vi "SIMCOMCommunicationTool_CF.vi"(0 "VISA资源名称":refnum<visa-resource-name>="COM26", 1 "MSComm":refnum<k7>, 2 "MEID":string, 5 "通信协议名称":string, 9 "DelayTime":u32=100, 11 "error in":errorcluster, 12 "Debug":bool=TRUE, 14 "Slot":T1) -> (3 "CMD":string="发送 重启:AT+CRESET\r反馈:\r\nOK\r\n\r\n", 4 "字符串数值":bool=TRUE, 6 "反馈结果":bool=TRUE, 10 "ReturnData":string, 15 "error out":errorcluster)   [LabVIEW 2013]
doc: "本范例根据用户指示，对串口执行读写操作。范例运行时可按下“写入”或“读取”按钮，以及修改“读数”。\n\n设置的串口参数必须匹配连接仪器或设备的参数。本范例中，“读数”参数可指定串口读取的字节数。如端口字节超过指定的字节数，超出部分将不会被读取。如端口字节数少于指定的字节数，将返回超时错误。\n\n本范例可扩展流控制选项以包括XON和XOFF，从而允许用户选择控制字符。同时，用户可启用或禁用中止符。部分设备需要通过终止符确定命令字符串的结束位置。部分设备将发送终止符以说明待读取数据的末端。本范例演示了缓冲区中检测到终止符时，结束“读取”操作或添加终止符至“写入”数据末端的方法。"
uses:
  SystemCode/SysControl/Slot.ctl
  <vilib>/Utility/NIReport.llb/NI_report.lvclass
  SourceCode/GlobalValue.vi
  <vilib>/Utility/error.llb/Error Cluster From Error Code.vi
  <vilib>/addons/_office/excel.llb/Excel Get Data ([str]).vi
  <vilib>/ErrorRing/Error Ring.xnode
  <vilib>/addons/_office/NI_ReportGenerationToolkit.lvlib
  <vilib>/Utility/NIReport.llb/Excel/NI_Excel.lvclass
panel:
  out "Data":string[][](array[string])=[["8986031490021881534", "460036161669975", "2A645416CB435F94", "8006A127", "460036161669975@mycdma.cn", "DB60264368A1D188", "18101891253", "A1000021A59070"], ["8986031490021881535", "460036161669976", "32FA5764D69C76BE", "80FAE4E6", "460036161669976@mycdma.cn", "B3AA1B3D2F0D5593", "18964872399", "A1000021A58D61"], ["", "", "", "", "", "", "", ""], ["", "", "", "", "", "", "", ""], ["", "", "", "", "", "", "", ""], ["", "", "", "", "", "", "", ""], ["", "", "", "", "", "", "", ""], ["", "", "", "", "", "", "", ""], ["", "", "", "", "", "", "", ""], ["", "", "", "", "", "", "", ""], ["", "各位，模块烧号主要是写五码，包括IMSI、AKEY、MEID（ESN）、AN(EVDO USER)、AAA(EVDO PWD)。", "", "", "", "", "", ""], ["", "其中ESN和MEID在模块出厂时已经写入，两者均可通过AT指令读取，但ESN不可更改。", "", "", "", "", "", ""], ["", "经询问及实际测试，上海电信绑定ESN号而广东电信未绑定，意味着上海电信五码烧录到其它模块是不可用的，但广东电信则无此限制。", "", "", "", "", "", ""], ["", "", "", "", "", "", "", ""], ["", "", "", "", "", "", "", ""], ["", "目前已确定跟上海电信合作，后续模块及卡号使用过程中，如遇到模块损坏，则意味着该卡必须销号（除非向电信申请绑定新的ESN），否则烧录到其它模块中是没用的。", "", "", "", "", "", ""]]
  in  "命令列表":u16(ring)=18 items=["查询RTRECF", "设置RTRECF", "查询MEID", "设置MEID", "查询ESN", "设置ESN", "查询AKEY", "设置AKEY", "查询IMSI1", "设置IMSI1", "查询IMSI2", "设置IMSI2", "查询IMSI3", "设置IMSI3", "设置EVDO账号", "设置EVDO密码", "打开音频LOOPBACK", "关闭音频LOOPBACK", "重启", "打开网络", "查询网络状态", "连网测试", "查询CIP", "切换声音通道", "测试登录", "拨号", "挂断", "查询IP", "AT+CSOCKAUTHNV", "AT+CSOCKAUTH", "查询2G信号", "查询3G信号", "H330测试通讯", "H330打开音频回环", "H330关闭音频回环", "H330拨号"]
  out "ConfigPath":string="D:\\导航\\T-BOX\\新建文件夹\\config\\通信协议.xls"
  out "DataType":string="AT+CRESET"
  out "命令":string="AT+CRESET\r"
  out "响应":string="\r\nOK\r\n"
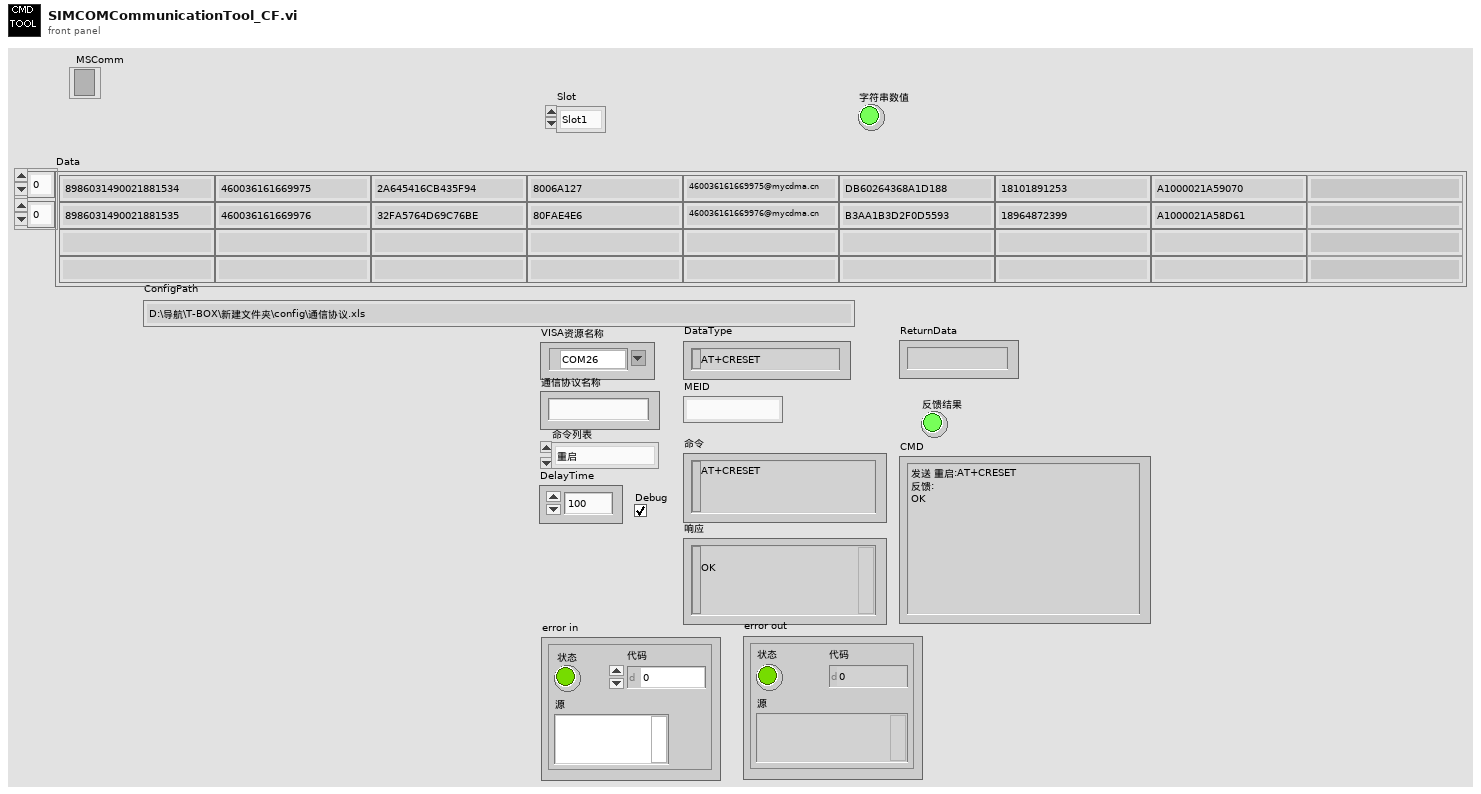
[diagram p1: front panel]
types:
  T1 = typedef "Slot.ctl" = enum16{"Slot1", "Slot2", "Slot3", "Slot4"}
  T2 = enum32{"invalid app kind", "Development System", "Run Time System", "Student Edition", "Embedded LabVIEW", "Evaluation", "Custom"}
  T3 = enum16{"maximized", "minimized", "normal", "no change"}
  T4 = enum16{"Standard Report", "HTML", "Word", "Excel"}
  T5 = cluster{"IMSI":string, "AKEY":string, "ESN":string, "EVDO账号":string, "EVDO密码":string, "设备号":string}
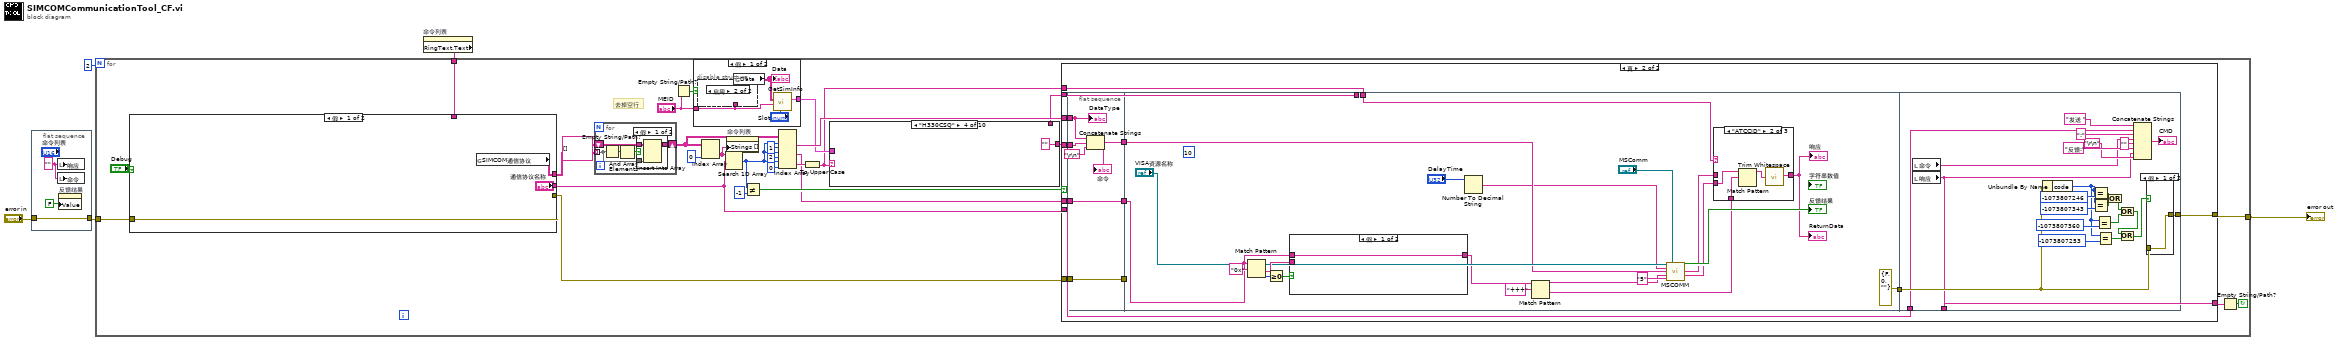
[diagram p0: block diagram]
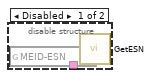
[diagram p2: hidden frame]
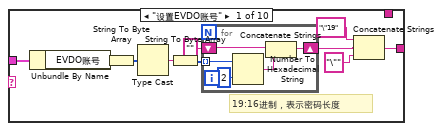
[diagram p5: hidden frame]
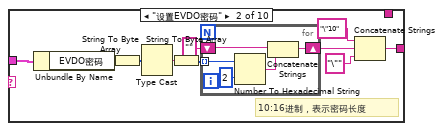
[diagram p6: hidden frame]
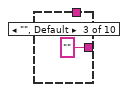
[diagram p7: hidden frame]
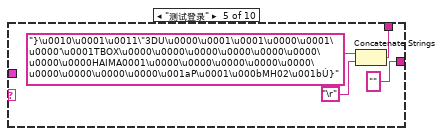
[diagram p8: hidden frame]
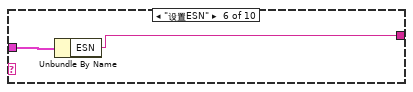
[diagram p9: hidden frame]
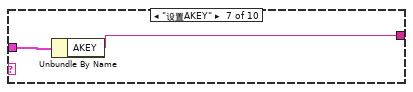
[diagram p10: hidden frame]
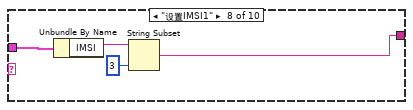
[diagram p11: hidden frame]
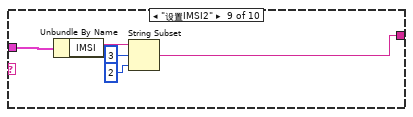
[diagram p12: hidden frame]
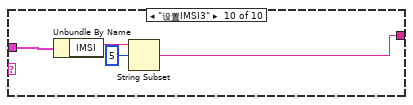
[diagram p13: hidden frame]
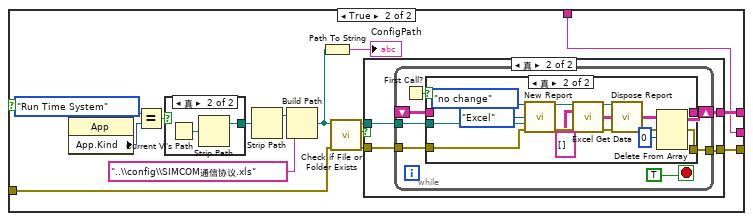
[diagram p14: hidden frame]
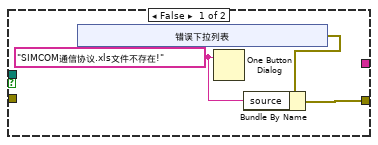
[diagram p15: hidden frame]
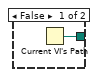
[diagram p17: hidden frame]
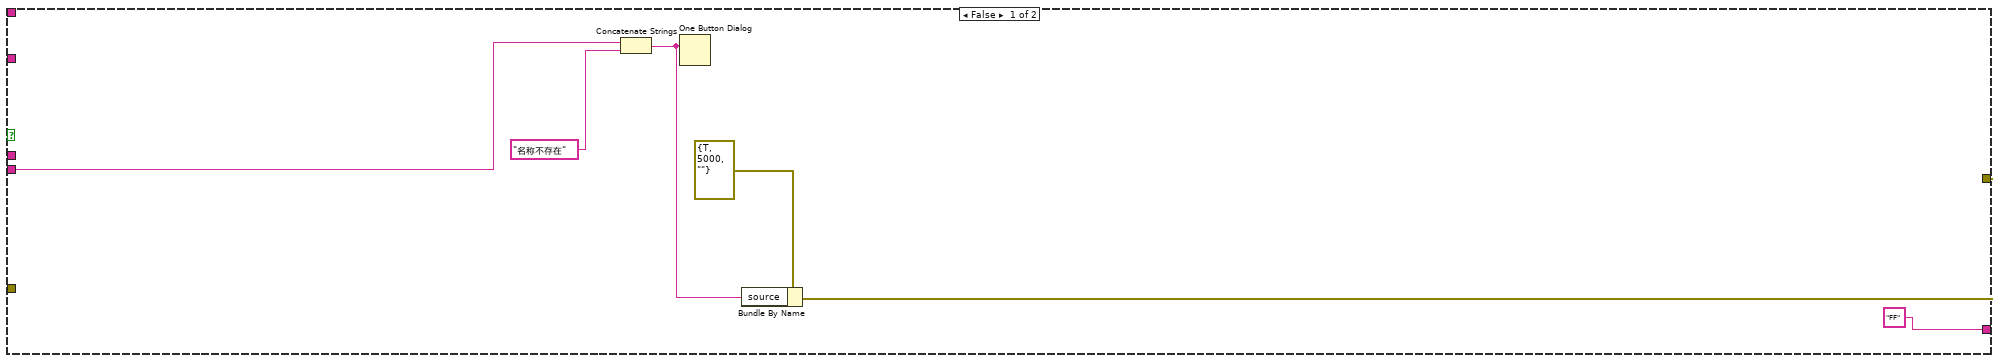
[diagram p18: hidden frame]
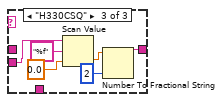
[diagram p20: hidden frame]
diagram:
  n1 = flat-sequence {
    tunnel: "error in" -> [w7]
    tunnel: [w7] -> w2
    frame #0 {
      w8 = "" ("响应")
      n2 = local write "响应"(w8) -> ()
      n3 = local write "命令"(w8) -> ()
      n4 = property on="反馈结果" class="Bool (严格)"("Value"=FALSE ("反馈结果")) -> ()  [unwired: 2 in, 2 out]
    }
  }
  n5 = property on="命令列表" class="Ring (严格)"() -> ("RingText.Text"=w1:string)  [unwired: 2 in, 2 out]
  n6 = for {
    N: 2 -> [_]
    tunnel: w2 -> [w24]
    tunnel: [w36] -> w5
    tunnel: w1 -> [w17]
    stop <- w22 continue-if-true
    # "去掉空行"
    n7 = case shown="假" "Debug" {
      tunnel: [w106 w111] -> w35
      tunnel: w24 -> [w106 w110]
      tunnel: ["通信协议名称" w108] -> w28
      tunnel: [w105 w109] -> w19
      tunnel: w17 -> [_ w108]
      frame False {
        n8 = global read "GlobalValue.vi" "SIMCOM通信协议"() -> (w105:string[][])
      }
      frame True {
        n9 = property class="App"() -> ("App.Kind"=w120:T2)  [unwired: 2 in, 2 out]
        n10 = Equal?(x=T2."Run Time System" ("y"), y=w120) -> (x = y?=w122:bool)
        n11 = case shown="真" w122 {
          tunnel: [w156 w158] -> w121
          frame False {
            n12 = Current VI's Path() -> (path=w156:path)
          }
          frame True {
            n13 = Current VI's Path() -> (path=w157:path)
            n14 = Strip Path(path=w157) -> (stripped path=w158:path)  [unwired: 1 out]
          }
        }
        n15 = Strip Path(path=w121) -> (stripped path=w115:path)  [unwired: 1 out]
        n16 = Build Path(base path=w115, name or relative path="..\\config\\SIMCOM通信协议.xls" ("连接的字符串")) -> (appended path=w117:path)
        n17 = Path To String(path=w117) -> (string=→"ConfigPath":string)
        n18 = call <vilib>:"Check if File or Folder Exists.vi"("error in (no error)"=w110, "path"=w117) -> ("error out"=w112:errorcluster, "file or folder exists?"=w114:bool, "dup path"=w113:path)  [unwired: 7 out]
        n19 = case shown="真" w114 {
          tunnel: w113 -> [_ w133]
          tunnel: w112 -> [_ w132]
          tunnel: [w124 w131] -> w111
          tunnel: [_ w130] -> w109
          frame False {
            w125 = "SIMCOM通信协议.xls文件不存在!" ("消息")
            n20 = xnode "错误下拉列表"() -> ("错误输出"=w123:errorcluster)
            n21 = One Button Dialog(message=w125) -> ()  [unwired: 1 in, 1 out]
            n22 = Bundle By Name(cluster=w123, "source"=w125) -> (w124:errorcluster)
          }
          frame True {
            n23 = while {
              tunnel: w133 -> [w139]
              tunnel: [w138] -> w131
              tunnel: w132 -> [w137]
              shift-right: [w140] -> w130
              shift-left: _ -> [w135]
              stop <- TRUE stop-if-true
              n24 = First Call?() -> (First Call?: T/F=w134:bool)
              n25 = case shown="真" w134 {
                tunnel: [w142 w146] -> w140
                tunnel: w139 -> [_ w145]
                tunnel: [w141 w144] -> w138
                tunnel: w137 -> [w141 w143]
                tunnel: w135 -> [w142 _]
                frame False {
                }
                frame True {
                  n26 = call <vilib>:"New Report.vi"("window state (normal)"=T3."no change", "report type"=T4."Excel", "template (empty)"=w145, "error in (no error)"=w143) -> ("report out"=w151:refnum<class "NI_report.lvclass">, "error out"=w152:errorcluster)  [unwired: 2 in, 8 out]
                  n27 = call-poly <vilib>:"Excel Get Data.vi"("report in"=w151, "data type"=string[][] [], "error in (no error)"=w152) -> ("report out"=w148:refnum<class "NI_report.lvclass">, "data"=w153:string[][], "error out"=w147:errorcluster)  [unwired: 10 in]
                  n28 = call-dynamic "Dispose Report.vi"("report in"=w148, "error in (no error)"=w147) -> ("error out"=w144:errorcluster)  [unwired: 3 in, 10 out]
                  n29 = Delete From Array(array=w153, index (row)=0 ("索引 (行)")) -> (array with subset deleted=w146:string[][])  [unwired: 2 in, 1 out]
                }
              }
            }
          }
        }
      }
    }
    n30 = for {
      tunnel: w19 -> [w43] mode=indexing
      shift-right: [w46] -> w18
      shift-left: string[][] [] -> [w47]
      n31 = Empty String/Path?(string/path=w43) -> (empty?=w45:bool[])
      n32 = And Array Elements(Boolean array=w45) -> (logical AND=w44:bool)
      n33 = case shown="假" w44 {
        tunnel: w47 -> [w50 w51]
        tunnel: [w49 w51] -> w46
        tunnel: w43 -> [w48 _]
        frame False {
          n34 = Insert Into Array(array=w50, new element=w48) -> (w49:string[][])  [unwired: 2 in]
        }
        frame True {
        }
      }
    }
    n35 = Empty String/Path?(string/path="MEID") -> (empty?=w10:bool)
    n36 = case shown="假" w10 {
      tunnel: [w40 _] -> w14
      tunnel: "MEID" -> [w37 _]
      frame False {
        n37 = disable-structure shown="启用" {
          disable-tunnel: w37 -> [w41 _]
          frame Disabled {
            n38 = global read "GlobalValue.vi" "MEID-ESN"() -> (w42:string[][])
            n39 = call "GetESN.vi"("MEID"=w41, "Data"=w42) -> ()  [unwired: 9 in, 1 out]
          }
          frame Enabled {
          }
        }
        n40 = global read "GlobalValue.vi" "Data"() -> (w39:string[][])
        "Data" <- w39
        n41 = call "GetSimInfo.vi"("Slot"="Slot", "MEID"=w37, "Data"=w39) -> ("SIMInfo"=w40:T5)  [unwired: 6 in, 2 out]
      }
      frame True {
      }
    }
    n42 = Index Array(array=w18, index (col)=0 ("禁用的索引 (列)")) -> (element=w26:string[])  [unwired: 1 in]
    n43 = Search 1D Array(1D array=w26, element=w28) -> (index of element=w21:i32)  [unwired: 1 in]
    n44 = property on="命令列表" class="Ring (严格)"("Strings []"=w26) -> ()  [unwired: 2 in, 2 out]
    n45 = Not Equal?(x=w21, y=-1) -> (x != y?=w30:bool)
    n46 = Index Array(array=w18, index (row) #1=w21, index (col) #1=1 ("索引 (列)"), index (row) #2=w21, index (col) #2=2 ("索引 (列)"), index (row) #3=w21, index (col) #3=0 ("索引 (列)")) -> (element #1=w15:string, element #2=w11:string, element #3=w16:string)
    n47 = To Upper Case(1:w16) -> (0:w12:string)
    n48 = case shown="\"H330CSQ\"" w12 {
      tunnel: [w54 w69 "" "" "" ("IMSI") w88 w90 w92 w97 w102] -> w29
      tunnel: w14 -> [w53 w67 _ _ _ w89 w91 w95 w100 w104]
      tunnel: [_ _ _ _ w84 _ _ _ _ _] -> w13
      frame "设置EVDO账号" {
        # "19:16进制，表示密码长度"
        n49 = Unbundle By Name(w53) -> ("EVDO账号"=w52:string)
        n50 = String To Byte Array(string=w52) -> (unsigned byte array=w61:u8[])
        n51 = Type Cast(x=w61) -> (*(type *) &x=w59:string)  [unwired: 1 in]
        n52 = String To Byte Array(string=w59) -> (unsigned byte array=w60:u8[])
        n53 = for {
          tunnel: w60 -> [w66] mode=indexing
          shift-right: [w64] -> w55
          shift-left: "" -> [w63]
          n54 = Number To Hexadecimal String(1:i16 2 ("宽度(-)"), 2:w66) -> (0:w65:string)
          n55 = Concatenate Strings(w63, w65) -> (w64:string)
        }
        n56 = Concatenate Strings("\"19" ("字符串"), w55, "\"" ("字符串")) -> (w54:string)
      }
      frame "设置EVDO密码" {
        # "10:16进制，表示密码长度"
        n57 = Unbundle By Name(w67) -> ("EVDO密码"=w68:string)
        n58 = String To Byte Array(string=w68) -> (unsigned byte array=w76:u8[])
        n59 = Type Cast(x=w76) -> (*(type *) &x=w74:string)  [unwired: 1 in]
        n60 = String To Byte Array(string=w74) -> (unsigned byte array=w75:u8[])
        n61 = for {
          tunnel: w75 -> [w81] mode=indexing
          shift-right: [w79] -> w72
          shift-left: "" -> [w78]
          n62 = Number To Hexadecimal String(1:i16 2 ("宽度(-)"), 2:w81) -> (0:w80:string)
          n63 = Concatenate Strings(w78, w80) -> (w79:string)
        }
        n64 = Concatenate Strings("\"10" ("字符串"), w72, "\"" ("字符串")) -> (w69:string)
      }
      frame "", Default {
      }
      frame "H330CSQ" {
      }
      frame "测试登录" {
        n65 = Concatenate Strings("}\u0010\u0001\u0011\"3DU\u0000\u0001\u0001\u0000\u0001\u0000'\u0001TBOX\u0000\u0000\u0000\u0000\u0000\u0000\u0000\u0000HAIMA0001\u0000\u0000\u0000\u0000\u0000\u0000\u0000\u0000\u0000\u001aP\u0001\u000bMH02\u001bÚ}" ("字符串"), "\r") -> (w84:string)
      }
      frame "设置ESN" {
        n66 = Unbundle By Name(w89) -> ("ESN"=w88:string)
      }
      frame "设置AKEY" {
        n67 = Unbundle By Name(w91) -> ("AKEY"=w90:string)
      }
      frame "设置IMSI1" {
        n68 = Unbundle By Name(w95) -> ("IMSI"=w94:string)
        n69 = String Subset(string=w94, length (rest)=3 ("长度（剩余）")) -> (substring=w92:string)  [unwired: 1 in]
      }
      frame "设置IMSI2" {
        n70 = Unbundle By Name(w100) -> ("IMSI"=w99:string)
        n71 = String Subset(string=w99, offset (0)=3 ("偏移量(0)"), length (rest)=2 ("长度（剩余）")) -> (substring=w97:string)
      }
      frame "设置IMSI3" {
        n72 = Unbundle By Name(w104) -> ("IMSI"=w103:string)
        n73 = String Subset(string=w103, offset (0)=5 ("偏移量(0)")) -> (substring=w102:string)  [unwired: 1 in]
      }
    }
    n74 = case shown="真" w30 {
      tunnel: w28 -> [w164 w170]
      tunnel: w15 -> [_ w177]
      tunnel: w29 -> [_ w176]
      tunnel: w35 -> [_ w175]
      tunnel: [w160 w173] -> w36
      tunnel: ["FF" ("响应") w172] -> w23
      tunnel: w13 -> [_ w169]
      tunnel: w12 -> [_ w168]
      tunnel: w11 -> [_ w167]
      frame False {
        n75 = Concatenate Strings(w164, "名称不存在" ("消息")) -> (w161:string)
        n76 = One Button Dialog(message=w161) -> ()  [unwired: 1 in, 1 out]
        n77 = Bundle By Name(cluster=errorcluster {"status"=TRUE, "code"=5000, "source"=""} ("error in 1 (no error)"), "source"=w161) -> (w160:errorcluster)
      }
      frame True {
        n78 = flat-sequence {
          tunnel: w177 -> [w182]
          tunnel: w176 -> [w181]
          tunnel: w175 -> [w183]
          tunnel: [w183] -> w174
          tunnel: [w180] -> w171
          tunnel: w167 -> [w178]
          tunnel: [w178] -> w166
          tunnel: w174 -> [_]
          tunnel: w171 -> [w198]
          tunnel: w169 -> [_]
          tunnel: w168 -> [w191]
          tunnel: w166 -> [w200]
          tunnel: [errorcluster {"status"=FALSE, "code"=0, "source"=""} ("错误输出")] -> w165
          tunnel: [w249] -> w173
          tunnel: w170 -> [w245]
          tunnel: [w239] -> w172
          tunnel: w165 -> [w248]
          frame #0 {
            n79 = Concatenate Strings(w182, w181, "\r\n") -> (w180:string)
            "命令" <- w180
            "DataType" <- w182
          }
          frame #1 {
            (unwired) 10
            n80 = Match Pattern(string=w200, regular expression="0x" ("正则表达式")) -> (after substring=w202:string, offset past match=w203:i32)  [unwired: 1 in, 2 out]
            n81 = Greater Or Equal To 0?(x=w203) -> (x >= 0?=w201:bool)
            n82 = case shown="假" w201 {
              tunnel: w202 -> [_ w218]
              tunnel: [w216 w217] -> w187
              tunnel: w200 -> [w216 _]
              frame False {
              }
              frame True {
                n83 = String Length(string=w218) -> (length=w221:i32)
                n84 = Divide(x=w221, y=2) -> (x/y=w219:dbl)
                n85 = for {
                  N: w219 -> [_]
                  tunnel: w218 -> [w227]
                  shift-right: [w229] -> w217
                  shift-left: "" -> [w228]
                  i -> [w225]
                  w223 = 2 ("x")
                  n86 = Multiply(x=w223, y=w225) -> (x*y=w224:i32)
                  n87 = String Subset(string=w227, offset (0)=w224, length (rest)=w223) -> (substring=w226:string)
                  n88 = Hexadecimal String To Number(string=w226) -> (number=w232:u32)  [unwired: 2 in, 1 out]
                  n89 = To Byte Integer(number=w232) -> (8bit integer=w231:i8)
                  n90 = Type Cast(x=w231) -> (*(type *) &x=w230:string)  [unwired: 1 in]
                  n91 = Concatenate Strings(w228, w230) -> (w229:string)
                }
              }
            }
            n92 = Number To Decimal String(number="DelayTime") -> (decimal integer string=w196:string)  [unwired: 1 in]
            n93 = Match Pattern(string=w187, regular expression="+++" ("正则表达式")) -> (before substring=w185:string, after substring=w184:string)  [unwired: 1 in, 2 out]
            n94 = call "MSCOMM.vi"("端口号"="VISA资源名称", "MSComm"="MSComm", "Send Delay(ms)"=w196, "Send Data"=w198, "Data Return"=w185, "cycle times"="5") -> ("result"=→"反馈结果":bool, "Rec Data"=w190:string, "Para"=w188:string)  [unwired: 7 in]
            n95 = case shown="\"ATCCID\"" w191 {
              tunnel: w190 -> [w205 _ _]
              tunnel: [w205 w207 w211] -> w189
              tunnel: w188 -> [_ w209 w214]
              tunnel: w184 -> [_ w208 _]
              frame "假", Default {
              }
              frame "ATCCID" {
                n96 = Match Pattern(string=w209, regular expression=w208) -> (before substring=w206:string)  [unwired: 1 in, 3 out]
                n97 = call <vilib>:"Trim Whitespace.vi"("string"=w206) -> ("trimmed string"=w207:string)  [unwired: 1 in]
              }
              frame "H330CSQ" {
                n98 = Scan Value(string=w214, format string="%f" ("格式字符串"), default (0 dbl)=0.0) -> (value=w212:dbl)  [unwired: 1 out]
                n99 = Number To Fractional String(number=w212, precision (6)=i16 2 ("精度(6)")) -> (F-format string=w211:string)  [unwired: 2 in]
              }
            }
            "ReturnData" <- w189
            "响应" <- w189
          }
          frame #2 {
            n100 = local read "命令"() -> (w240:string)
            n101 = local read "响应"() -> (w239:string)
            n102 = Unbundle By Name(w248) -> ("code"=w237:i32)
            n103 = Equal?(x=w237, y=-1073807246) -> (x = y?=w246:bool)
            n104 = Equal?(x=w237, y=-1073807343) -> (x = y?=w243:bool)
            n105 = Equal?(x=w237, y=-1073807360) -> (x = y?=w241:bool)
            n106 = Equal?(x=w237, y=-1073807253) -> (x = y?=w234:bool)
            n107 = Or(x=w246, y=w243) -> (x .or. y?=w242:bool)
            n108 = Or(x=w242, y=w241) -> (x .or. y?=w235:bool)
            n109 = Or(x=w235, y=w234) -> (x .or. y?=w233:bool)
            n110 = Concatenate Strings("发送 " ("字符串"), w245, ":" ("字符串"), w240, "" ("字符串"), "反馈:" ("字符串"), w239, "\r\n") -> (→"CMD":string)
            n111 = case shown="假" w233 {
              tunnel: [w256 errorcluster {"status"=FALSE, "code"=0, "source"=""} ("t")] -> w249
              tunnel: w248 -> [w256 _]
              frame False {
              }
              frame True {
              }
            }
          }
        }
      }
    }
    n112 = Empty String/Path?(string/path=w23) -> (empty?=w22:bool)
  }
  "error out" <- w5
